vi "Do Collision.vi"(9 "Team in":refnum<class "Team.lvclass">, 11 "Square":refnum<class "Square.lvclass">) -> (1 "Team out":refnum<class "Team.lvclass">)   [LabVIEW 2020, in "SquareBattle.lvlib" / "Square.lvclass"]
uses:
  Square.lvclass
  Team/Team.lvclass
  Team Stats.ctl
  SquareBattle.lvlib
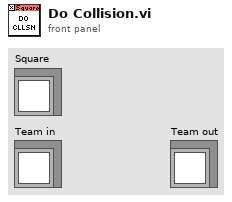
[diagram p1: front panel]
types:
  T1 = typedef "SquareBattle.lvlib/Team Stats.ctl" = cluster{"Active":i32, "Generated":i32, "Kills":i32, "Eliminated":i32, "Collided":i32}
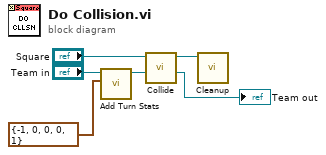
[diagram p0: block diagram]
diagram:
  n1 = call "Add Turn Stats.vi"("Team Stats"=T1 {"Active"=-1, "Generated"=0, "Kills"=0, "Eliminated"=0, "Collided"=1}, "Team in"="Team in") -> ("Team out"=w3:refnum<class "Team.lvclass">)  [unwired: 9 in]
  n2 = call-dynamic "Collide.vi"("Team In"=w3, "Square in"="Square") -> ("Team"=→"Team out":refnum<class "Team.lvclass">, "Square out"=w2:refnum<class "Square.lvclass">)  [unwired: 8 in]
  n3 = call-dynamic "Cleanup.vi"("Square"=w2) -> ()  [unwired: 11 in]
